vi "Two Sensor Test.vi"() -> ()   [LabVIEW 2013]
uses:
  <vilib>/FPGAPlugInAG/sbRIO-9642/niLvFpga_Open_sbRIO-9642.vi
  <vilib>/rvi/interface/common/dynamic/niFpgaDynamicAddResources.vi
  <vilib>/rvi/interface/common/niFpgaWaitOnOcc.vi
  <vilib>/Utility/error.llb/Error Cluster From Error Code.vi
  <vilib>/rvi/errors/niLvFpgaAdjustHostInterfaceError.vi
  <vilib>/rvi/interface/nirviOpenFPGA/nirviOpenFPGA.xnode
  FPGA Bitfiles/NatesProject1_FPGATarget_FPGAConfig_gDHlPw7zMRU.lvbitx
  FPGA Config.vi
  <vilib>/rvi/interface/nirviReadWriteControl/nirviReadWriteControl.xnode
  NiFpgaLv.dll
  <vilib>/rvi/interface/Simulation/niFpgaSimulationCallBeginRW.vi
panel:
  out "ModA/AI1":fxp<+/-,26,5>
  out "Front Sensor\nDistance\n(cm)":dbl(slide) scale=0.0..150.0
  out "Rear Sensor\nDistance\n(cm)":dbl(slide) scale=0.0..150.0
  in  "stop":bool
  out "ModA/AI0":fxp<+/-,26,5>
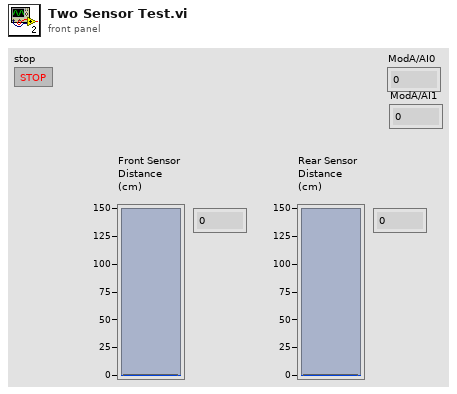
[diagram p1: front panel]
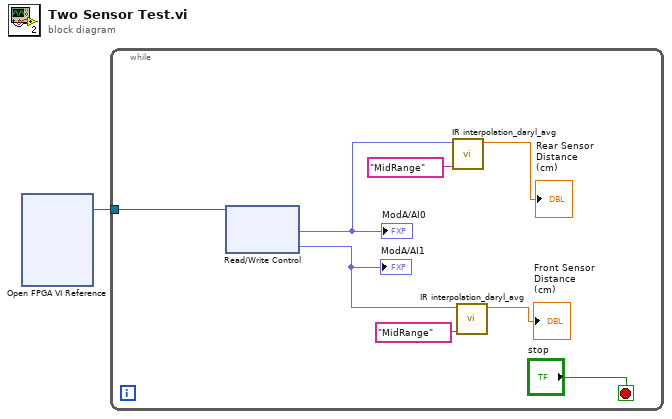
[diagram p0: block diagram]
diagram:
  n1 = xnode "Open FPGA VI Reference"() -> ("FPGA VI Reference Out"=w1:refnum<k20>)  [unwired: 2 in, 1 out]
  n2 = while {
    tunnel: w1 -> [w2]
    stop <- "stop" stop-if-true
    n3 = xnode "Read/Write Control"("FPGA VI Reference In"=w2) -> ("ModA/AI0"=w8:fxp<+/-,26,5>, "ModA/AI1"=w5:fxp<+/-,26,5>)  [unwired: 1 in, 2 out]
    "ModA/AI0" <- w8
    "ModA/AI1" <- w5
    n4 = call "IR interpolation_daryl_avg.vi"("IR Sensor Type"="MidRange", "x value"=w8) -> ("interpolation value"=→"Rear Sensor\nDistance\n(cm)":dbl)  [unwired: 9 in]
    n5 = call "IR interpolation_daryl_avg.vi"("IR Sensor Type"="MidRange", "x value"=w5) -> ("interpolation value"=→"Front Sensor\nDistance\n(cm)":dbl)  [unwired: 9 in]
  }
